vi "Request.vi"(5 "Response Type (None)":refnum<class>, 6 "Timeout ms (1000)":i32=1000, 7 "High Priority (F)":bool, 8 "error in (no error)":errorcluster, 9 "Data":variant, 10 "ID":string, 11 "MessageQ in":refnum<class "MessageQ.lvclass">) -> (0 "error out":errorcluster, 2 "Response":refnum<class>, 3 "MessageQ out":refnum<class "MessageQ.lvclass">)   [LabVIEW 2020, in "Volatus.lvlib" / "MessageQ.lvclass"]
uses:
  MessageQ.lvclass
  Request Message.ctl
  lv-promises/Promises/Promise/Promise.lvclass
  lv-promises/Promises/Promise/Promise.lvclass/Promise.ctl
  lv-promises/Promises/Future/Future.lvclass/Future.ctl
  MessageQ.lvclass/MessageQ.ctl
  lv-promises/Promises/Future/Future.lvclass
  Volatus.lvlib
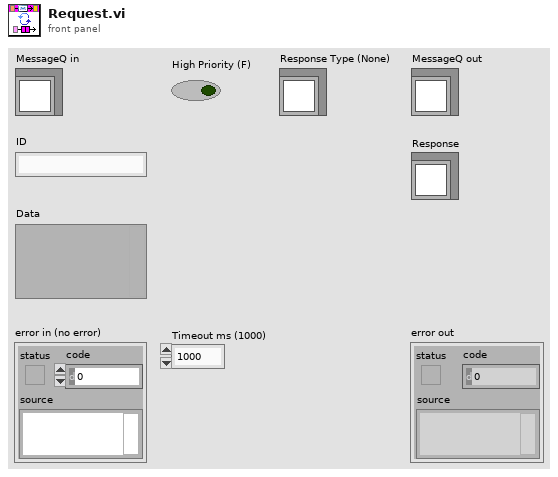
[diagram p1: front panel]
types:
  T1 = typedef "Volatus.lvlib/Request Message.ctl" = cluster{"Promise":refnum<class "Promise.lvclass">, "Data":variant}
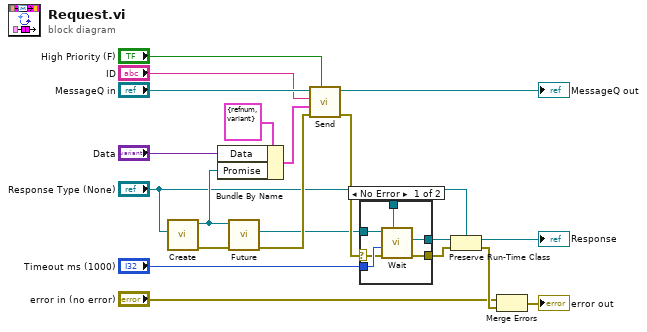
[diagram p0: block diagram]
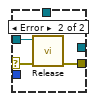
[diagram p2: hidden frame]
diagram:
  n1 = call "Create.vi"("Result Type (Variant)"="Response Type (None)") -> ("error out"=w18:errorcluster, "Promise"=w10:refnum<class "Promise.lvclass">)  [unwired: 9 in]
  n2 = Bundle By Name(cluster=T1 {"Promise"=refnum, "Data"=variant} ("Request Message"), "Data"="Data", "Promise"=w10) -> (w11:T1)
  n3 = call "Future.vi"("Promise in"=w10) -> ("Future"=w9:refnum<class "Future.lvclass">)  [unwired: 9 in, 1 out]
  n4 = call "Send.vi"("High Priority (F)"="High Priority (F)", "error in (no error)"=w18, "Data"=w11, "ID"="ID", "MessageQ in"="MessageQ in") -> ("error out"=w19:errorcluster, "MessageQ out"=→"MessageQ out":refnum<class "MessageQ.lvclass">)  [unwired: 5 in]
  n5 = case shown="No Error" w19 {
    selector: w19 -> [w22 w26]
    tunnel: w9 -> [w25 w27]
    tunnel: "Response Type (None)" -> [w24 _]
    tunnel: "Timeout ms (1000)" -> [w23 _]
    tunnel: [w21 _] -> w7
    tunnel: [w20 w26] -> w5
    frame No Error {
      n6 = call "Wait.vi"("Result Type (Variant)"=w24, "error in (no error)"=w22, "Timeout mS (-1)"=w23, "Future in"=w25) -> ("error out"=w20:errorcluster, "Result"=w21:refnum<class>)  [unwired: 6 in]
    }
    frame Error {
      n7 = call "Release.vi"("Future in"=w27) -> ()  [unwired: 11 in]
    }
  }
  n8 = Preserve Run-Time Class(object in=w7, error in=w5, 2:"Response Type (None)") -> (object out=→"Response":refnum<class>, error out=w3:errorcluster)
  n9 = Merge Errors("error in (no error)", w3) -> (→"error out":errorcluster)
